vi "PDA_RegMode_Acquisition.vi"(4 "Shutter":bool=TRUE, 5 "error in":errorcluster, 6 "StartIng Mode":T1(ring)=enum."Reset", 7 "Number of Cycles":u32=1 min=1 max=30, 8 "Acquisition Parameters":T2={"Exposure (ms)"=100, "Interval (ms)"=10, "Flush Count"=1, "Trigger"=0} {"Trigger" items=["Disable", "Acquistion", "Cycle"]}) -> (0 "error out":errorcluster, 1 "# Pixel Overflow":i32, 2 "PDA Overflow":bool, 3 "Output Array":dbl[](array[numeric]) format="%.2f")   [LabVIEW 2019]
doc: "This VI demonstrates acquisition and image display of CCD data\nutilizing the ISA CCD driver.\n\nNote: Specific help is available for each individual control, display and indicator."
uses:
  Globals and TypeDefs/Type Definitions.llb/3 way Status.ctl
  Globals and TypeDefs/gStatus.vi
  IGA_comm.llb/Controller Version Number.vi
panel:
  out "PDA Temperature after":dbl
  out "Temperature":dbl
  in  "Tab Control":enum32{"Original Signals", "Averaged Output"}(tab)
  out "Display":sgl[][](graph)
  out "Display 2":dbl[](graph)
  out "Current Operation":T1(ring)
  in  "Gain":bool
  out "Read # count":u32=1 min=1 max=30
  in  "Number of Region copy":u32=4
  in  "Number of Regions":u32=1
  out "Acq Busy":bool
  # "Before        After"
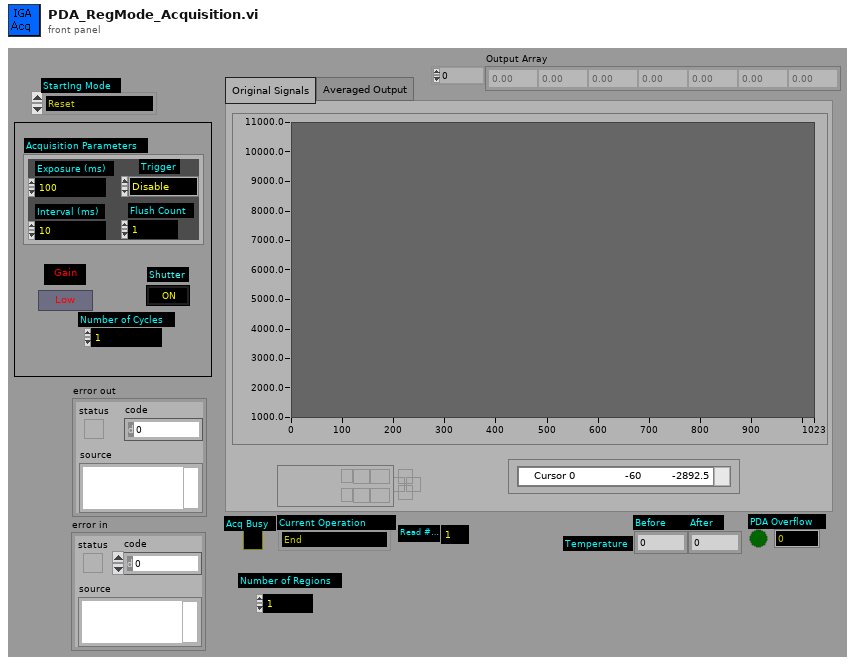
[diagram p1: front panel]
types:
  T1 = enum16{"End", "Init", "Reset", "SetAcqParameter", "SetArea", "Start Acquisition", "Busy Status Poll", "Read", "Stop"}
  T2 = cluster{"Exposure (ms)":u32, "Interval (ms)":u32, "Flush Count":i32, "Trigger":u16}
  T3 = typedef "3 way Status.ctl" = u8
  T4 = cluster{"Comm Interface":u16, "BUS":i16, "Address":i16, "Com Port":i32}
  T5 = enum16{"CCD Temperature Z345", "CCD Temperature Z308", "CCD Gain"}
  T6 = enum16{"Motor Init", "Motor Set Speed", "Motor Read Speed", "Motor Go", "Motor Busy Check", "Motor Move Relative", "Motor Set Position", "Motor Read Position", "Threshold Write Value", "Threshold Read Values", "Motor Limit Status", "Motor Stop", "ACQ Start", "ACQ Stop", "ACQ Integration Time Set", "ACQ Integration Time Read", "ACQ Busy", "ACQ Channel Gain Set", "ACQ Gain Read", "ACQ Read Data", "High Voltage Set", "High Voltage Read", "ACC Shutter Open", "ACC Shutter Close", "ACC Turret Position 1", "ACC Turret Position 0", "ACC ENTR Mirror Side", "ACC ENTR Mirror Front", "ACC Exit Mirror Side", "ACC Exit Mirror Front", "Slit Set Speed", "Slit Read Speed", "Slit Set Position", "Slit Read Position", "Slit Move Relative", "ACC Busy Check", "TTL Write Output", "TTL Read Output", "TTL Read Input", "Scan Set Parameters", "Scan Start", "Scan Current Status", "Scan Cycle to Read", "Scan Get Data Point Number", "Scan Get Data", "Scan Stop", "ACQ Measure Offsets", "ACQ Set Offsets", "TTL Automatic Outputs", "CCD_INIT", "CCD_SET_EXPOSURE_TIME", "CCD_SET_GAIN", "CCD_READ_GAIN", "CCD_SET_NUMBER_OF_FLUSHES", "CCD_SET_DOUBLE_COR_TIME", "CCD_SET_TEMPERATURE", "CCD_READ_TEMPERATURE", "CCD_READ_CHIP_STUFF", "CCD_START", "CCD_STATUS", "CCD_STOP", "CCD_READ_IMAGE", "CCD_READ_SCAN", "CCD_RESET_IMAGE", "CCD_READ_NEXT_SCAN", "CCD_RESET_SCAN", "CCD_SET_SHUTTER", "CCD_DEFINE_ACQ_FORMAT", "CCD_DEFINE_AREA", "CCD_GET_DATA_SIZE", "CCD_WRITE_CHIP_STUFF", "CCD_GO_BLAST", "CCD_TRIGGER_ENABLE", "CCD_SET_BLAST_INTERVAL", "CCD_WRITE_XDATA", "CCD_READ_XDATA", "CCD_STUFF_XDATA", "CCD_SET_MUX_AND_READ_ADC", "CCD_SET_SPEED_FACTOR", "CCD_SET_FLUSH_MODE", "CCD_GET_READOUT_TIME", "CCD Go ICCD", "CCD Select ADC"}
  T7 = cluster{"X Origin":u32, "Y Origin":u32, "X Size":u32, "Y Size":u32, "X Bin":u32, "Y Bin":u32}[]
  T8 = cluster{"Exposure (ms)":bool, "Interval (ms)":bool, "Flush Count":bool, "Trigger":bool}
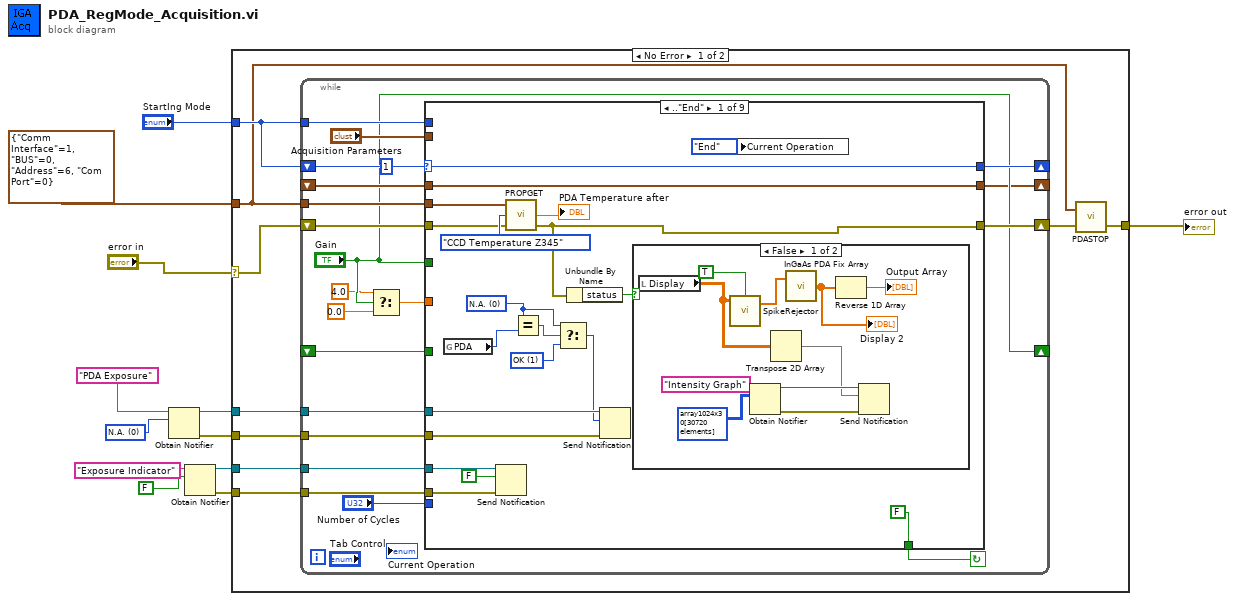
[diagram p0: block diagram]
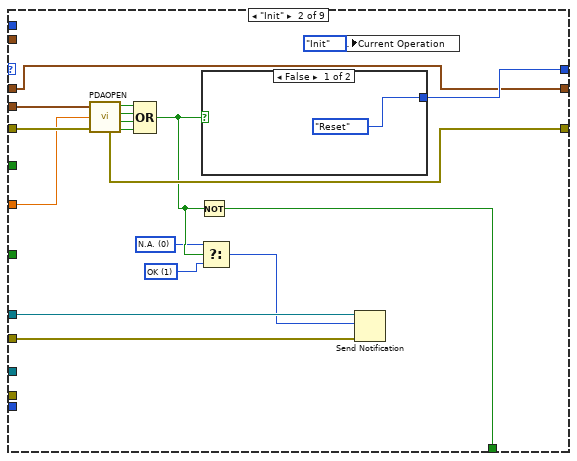
[diagram p3: hidden frame]
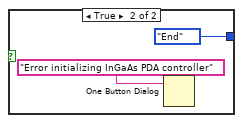
[diagram p4: hidden frame]
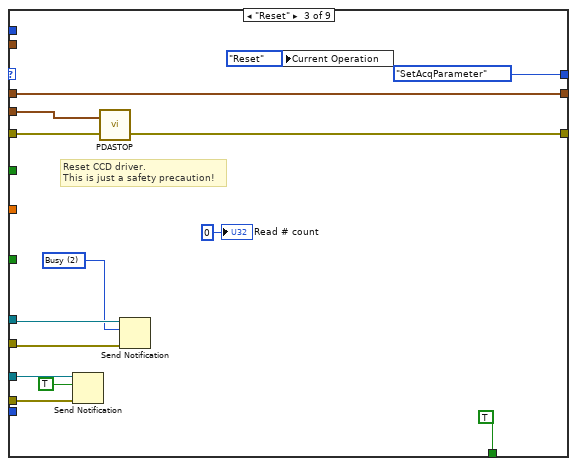
[diagram p5: hidden frame]
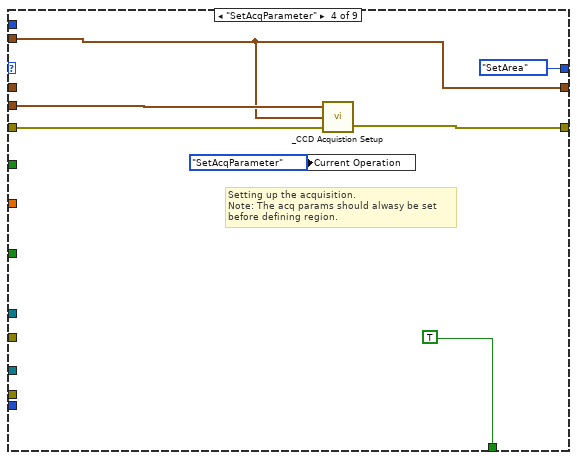
[diagram p6: hidden frame]
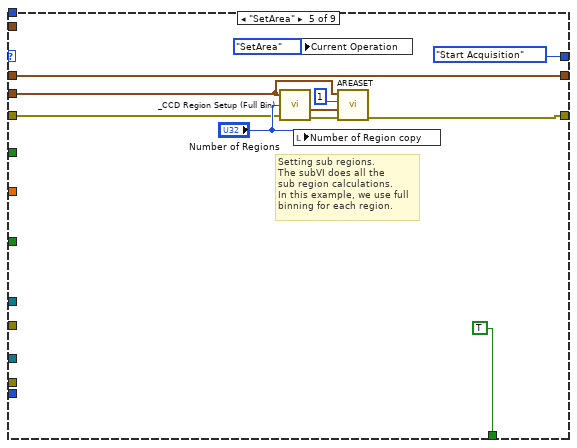
[diagram p7: hidden frame]
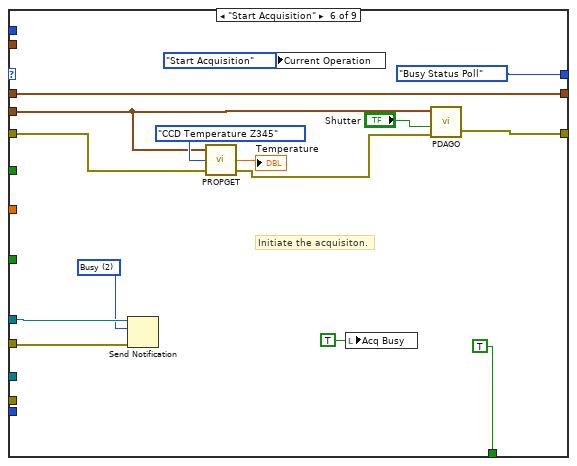
[diagram p8: hidden frame]
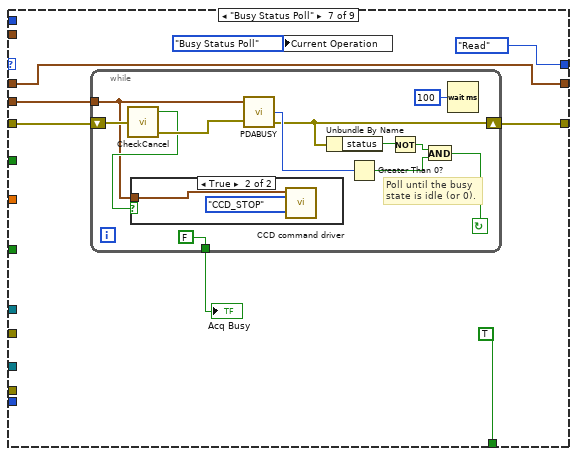
[diagram p9: hidden frame]
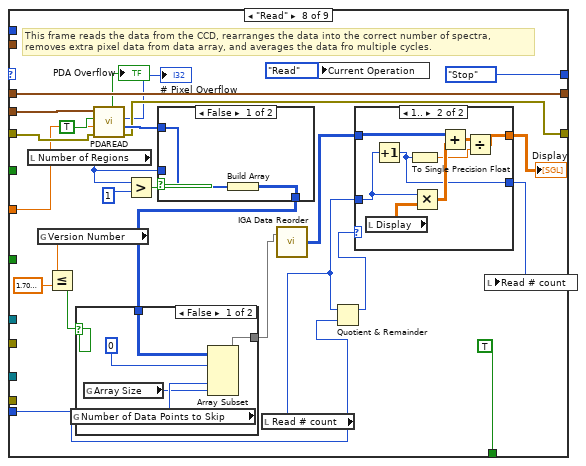
[diagram p11: hidden frame]
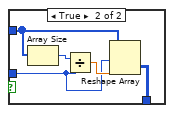
[diagram p13: hidden frame]
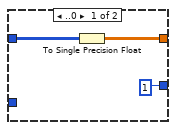
[diagram p14: hidden frame]
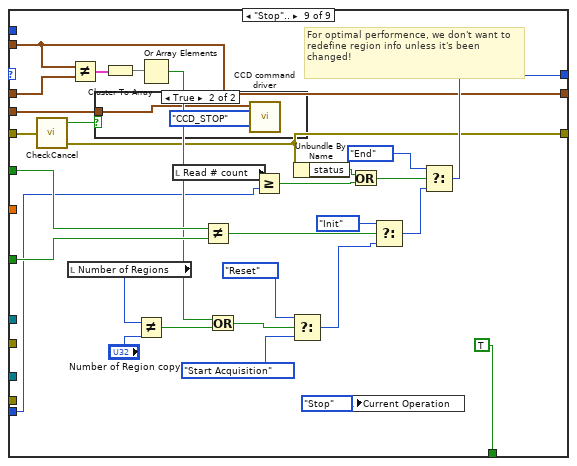
[diagram p15: hidden frame]
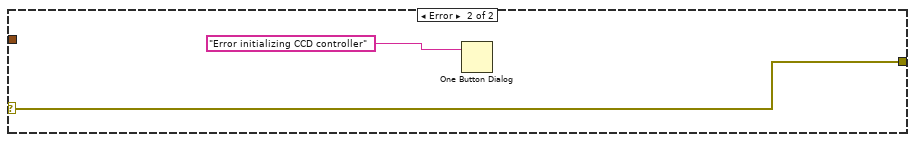
[diagram p17: hidden frame]
diagram:
  w8 = T3 0 items=["N.A.", "OK", "Busy", "Done"] ("Saving")
  n1 = Obtain Notifier(name (unnamed)="PDA Exposure", notification data type=w8) -> (notifier out=w7:refnum<notifier>, error out=w6:errorcluster)  [unwired: 2 in, 1 out]
  n2 = Obtain Notifier(name (unnamed)="Exposure Indicator", notification data type=FALSE ("SaveData?")) -> (notifier out=w3:refnum<notifier>, error out=w2:errorcluster)  [unwired: 2 in, 1 out]
  n3 = case shown="No Error" "error in" {
    selector: "error in" -> [w21 w244]
    tunnel: T4 {"Comm Interface"=1, "BUS"=0, "Address"=6, "Com Port"=0} ("Comm Params") -> [w17 _]
    tunnel: "StartIng Mode" -> [w19 _]
    tunnel: [w18 w244] -> w10
    tunnel: w7 -> [w16 _]
    tunnel: w6 -> [w15 _]
    tunnel: w3 -> [w14 _]
    tunnel: w2 -> [w13 _]
    frame No Error {
      (unwired) 1
      n4 = while {
        shift-left: w21 -> [w39]
        shift-right: [w40] -> w20
        tunnel: w17 -> [w38]
        shift-right: [w27] -> _
        shift-left: _ -> [w37]
        tunnel: w19 -> [w36]
        shift-right: ["Gain"] -> _
        shift-left: _ -> [w35]
        shift-right: [w34] -> _
        shift-left: w19 -> [w33]
        tunnel: w16 -> [w25]
        tunnel: w15 -> [w24]
        tunnel: w14 -> [w23]
        tunnel: w13 -> [w22]
        stop <- w41 continue-if-true
        n5 = Select(t=4.0, s="Gain", f=0.0) -> (s? t:f=w30:dbl)
        n6 = case shown="..\"End\"" w33 {
          selector: w33 -> [w60 _ _ _ _ _ _ _ _]
          tunnel: [FALSE w83 TRUE TRUE TRUE TRUE TRUE TRUE TRUE] -> w41
          tunnel: [w60 w81 T1."SetAcqParameter" ("StartIng Mode") T1."SetArea" ("StartIng Mode") T1."Start Acquisition" ("StartIng Mode") T1."Busy Status Poll" ("StartIng Mode") T1."Read" ("StartIng Mode") T1."Stop" ("StartIng Mode") w238] -> w34
          tunnel: w39 -> [w51 w85 w104 w111 w115 w127 w146 w170 w215]
          tunnel: [w49 w82 w103 w110 w118 w137 w144 w169 w214] -> w40
          tunnel: "Gain" -> [_ _ _ _ _ _ _ _ w234]
          tunnel: w38 -> [w50 w84 w102 w112 w119 w125 w145 w171 w212]
          tunnel: w37 -> [w59 w79 w101 _ w117 w134 w141 w166 w223]
          tunnel: w36 -> [_ _ _ _ _ _ _ _ _]
          tunnel: w35 -> [_ _ _ _ _ _ _ _ w233]
          tunnel: "Acquisition Parameters" -> [_ _ _ w108 _ _ _ _ w220]
          tunnel: w30 -> [_ w80 _ _ _ _ _ w167 _]
          tunnel: [w59 w79 w101 w108 w117 w134 w141 w166 w220] -> w27
          tunnel: "Number of Cycles" -> [_ _ _ _ _ _ _ w164 w217]
          tunnel: w25 -> [w57 w77 w98 _ _ w132 _ _ _]
          tunnel: w24 -> [w56 w76 w97 _ _ w131 _ _ _]
          tunnel: w23 -> [w44 _ w95 _ _ _ _ _ _]
          tunnel: w22 -> [w43 _ w94 _ _ _ _ _ _]
          frame .."End" {
            w45 = T3 0 items=["N.A.", "OK", "Busy", "Done"] ("x")
            w55 = T3 1 items=["N.A.", "OK", "Busy", "Done"] ("Saving")
            n7 = global read "gStatus.vi" "PDA"() -> (w47:T3)
            n8 = Send Notification(notification=FALSE, notifier=w44, error in (no error)=w43) -> ()  [unwired: 2 out]
            n9 = call "PROPGET.VI"("error in"=w51, "CCD Prop ID"=T5."CCD Temperature Z345", "Comm Params"=w50) -> ("error out"=w49:errorcluster, "Output Param"=→"PDA Temperature after":dbl)  [unwired: 1 out]
            n10 = Equal?(x=w45, y=w47) -> (x = y?=w46:bool)
            n11 = Select(t=w45, s=w46, f=w55) -> (s? t:f=w54:T3)
            n12 = Unbundle By Name(w49) -> ("status"=w48:bool)
            n13 = Send Notification(notification=w54, notifier=w57, error in (no error)=w56) -> ()  [unwired: 2 out]
            n14 = case shown="False" w48 {
              frame False {
                n15 = local read "Display"() -> (w63:sgl[][])
                n16 = call "SpikeRejector.vi"("Average Only (T)"=TRUE, "Input Array"=w63) -> ("Final Array"=w71:dbl[])  [unwired: 2 in, 1 out]
                n17 = Obtain Notifier(name (unnamed)="Intensity Graph", notification data type=i32[][] array1024x30[30720 elements] ("Intensity Graph")) -> (notifier out=w66:refnum<notifier>, error out=w67:errorcluster)  [unwired: 2 in, 1 out]
                n18 = Transpose 2D Array(2D array=w63) -> (transposed array=w62:sgl[][])
                n19 = call "InGaAs PDA Fix Array.vi"("Input Array"=w71) -> ("Output Array"=w69:dbl[])  [unwired: 2 in]
                "Display 2" <- w69
                n20 = Reverse 1D Array(array=w69) -> (reversed array=→"Output Array":dbl[])
                n21 = Send Notification(notification=w62, notifier=w66, error in (no error)=w67) -> ()  [unwired: 2 out]
              }
              frame True {
              }
            }
            n22 = local write "Current Operation"(T1."End" ("Current Operation")) -> ()
          }
          frame "Init" {
            w73 = T3 1 items=["N.A.", "OK", "Busy", "Done"] ("Saving")
            w74 = T3 0 items=["N.A.", "OK", "Busy", "Done"] ("Saving")
            n23 = call "PDAOPEN.VI"("error in"=w85, "CCD ADC and Gain"=w80, "Comm Params"=w84) -> ("State Error"=w86:bool, "error out"=w82:errorcluster, "Table Error"=w87:bool, "Init Error"=w88:bool, "Boot Error"=w89:bool)  [unwired: 1 out]
            n24 = Compound Arithmetic op=OR(w89, w88, w87, w86) -> (w75:bool)
            n25 = Not(x=w75) -> (.not. x?=w83:bool)
            n26 = Select(t=w74, s=w75, f=w73) -> (s? t:f=w72:T3)
            n27 = case shown="False" w75 {
              tunnel: [T1."Reset" ("StartIng Mode") T1."End" ("StartIng Mode")] -> w81
              frame False {
              }
              frame True {
                n28 = One Button Dialog(message="Error initializing InGaAs PDA controller") -> ()  [unwired: 1 in, 1 out]
              }
            }
            n29 = local write "Current Operation"(T1."Init" ("Current Operation")) -> ()
            n30 = Send Notification(notification=w72, notifier=w77, error in (no error)=w76) -> ()  [unwired: 2 out]
          }
          frame "Reset" {
            w96 = T3 2 items=["N.A.", "OK", "Busy", "Done"] ("notification")
            # "Reset CCD driver.\nThis is just a safety precaution!"
            n31 = Send Notification(notification=TRUE, notifier=w95, error in (no error)=w94) -> ()  [unwired: 2 out]
            n32 = call "PDASTOP.VI"("error in"=w104, "Comm Params"=w102) -> ("error out"=w103:errorcluster)  [unwired: 1 out]
            n33 = Send Notification(notification=w96, notifier=w98, error in (no error)=w97) -> ()  [unwired: 2 out]
            n34 = local write "Current Operation"(T1."Reset" ("Current Operation")) -> ()
            "Read # count" <- u32 0 ("Read count")
          }
          frame "SetAcqParameter" {
            # "Setting up the acquisition.\nNote: The acq params should alwasy be set\nbefore defining region."
            n35 = local write "Current Operation"(T1."SetAcqParameter" ("Current Operation")) -> ()
            n36 = call "_CCD Acquistion Setup.vi"("error in"=w111, "Acquisition Param"=w108, "Comm Params"=w112) -> ("error out"=w110:errorcluster)  [unwired: 1 out]
          }
          frame "SetArea" {
            # "Setting sub regions.\nThe subVI does all the\nsub region calculations.\nIn this example, we use full\nbinning for each region."
            n37 = call "_CCD Region Setup (Full Bin).vi"("Comm Params"=w119, "Number of Regions"="Number of Regions", "error in"=w115) -> ("Region Info Array"=w122:T7, "error out"=w114:errorcluster)  [unwired: 2 out]
            n38 = local write "Number of Region copy"("Number of Regions") -> ()
            n39 = local write "Current Operation"(T1."SetArea" ("Current Operation")) -> ()
            n40 = call "AREASET.VI"("error in"=w114, "Region Info Array"=w122, "Acquisition Format"=1, "Comm Params"=w119) -> ("error out"=w118:errorcluster)  [unwired: 3 in, 1 out]
          }
          frame "Start Acquisition" {
            w130 = T3 2 items=["N.A.", "OK", "Busy", "Done"] ("notification")
            # "Initiate the acquisiton."
            n41 = Send Notification(notification=w130, notifier=w132, error in (no error)=w131) -> ()  [unwired: 2 out]
            n42 = call "PROPGET.VI"("error in"=w127, "CCD Prop ID"=T5."CCD Temperature Z345", "Comm Params"=w125) -> ("error out"=w126:errorcluster, "Output Param"=→"Temperature":dbl)  [unwired: 1 out]
            n43 = local write "Current Operation"(T1."Start Acquisition" ("Current Operation")) -> ()
            n44 = local write "Acq Busy"(TRUE ("Acq Busy")) -> ()
            n45 = call "PDAGO.VI"("error in"=w126, "Shutter"="Shutter", "Comm Params"=w125) -> ("error out"=w137:errorcluster)  [unwired: 1 in, 1 out]
          }
          frame "Busy Status Poll" {
            n46 = while {
              shift-right: [w157] -> w144
              shift-left: w146 -> [w151]
              tunnel: w145 -> [w148]
              tunnel: [FALSE ("Acq Busy")] -> w142
              stop <- w153 continue-if-true
              # "Poll until the busy\nstate is idle (or 0)."
              n47 = call "CheckCancel.vi"("error in (no error)"=w151) -> ("Cancelled"=w149:bool, "error out"=w150:errorcluster)  [unwired: 1 in]
              n48 = case shown="True" w149 {
                tunnel: w148 -> [_ w160]
                frame False {
                }
                frame True {
                  n49 = call "CCD command driver.VI"("Command"=T6."CCD_STOP", "Comm Params"=w160) -> ()  [unwired: 5 in, 5 out]
                }
              }
              n50 = call "PDABUSY.VI"("Comm Params"=w148, "error in"=w150) -> ("CCD Status"=w159:u16, "error out"=w157:errorcluster)  [unwired: 1 out]
              n51 = Unbundle By Name(w157) -> ("status"=w156:bool)
              n52 = Greater Than 0?(x=w159) -> (x > 0?=w154:bool)
              n53 = Not(x=w156) -> (.not. x?=w155:bool)
              n54 = And(x=w155, y=w154) -> (x .and. y?=w153:bool)
              n55 = Wait (ms)(milliseconds to wait=u32 100) -> ()  [unwired: 1 out]
            }
            "Acq Busy" <- w142
            n56 = local write "Current Operation"(T1."Busy Status Poll" ("Current Operation")) -> ()
          }
          frame "Read" {
            # "This frame reads the data from the CCD, rearranges the data into the correct number of spectra, \nremoves extra pixel data from data array, and averages the data fro multiple cycles."
            n57 = local read "Number of Regions"() -> (w182:u32)
            n58 = global read "Controller Version Number.vi" "Version Number"() -> (w177:sgl)
            n59 = Less Or Equal?(x=w177, y=sgl 1.7) -> (x <= y?=w175:bool)
            n60 = call "PDAREAD.VI"("Comm Params"=w171, "Reset Image?"=TRUE, "CCD ADC and Gain"=w167, "error in"=w170) -> ("PDA Overflow"=→"PDA Overflow":bool, "Pixel Overflow"=→"# Pixel Overflow":i32, "Data"=w181:u16[], "error out"=w169:errorcluster)  [unwired: 1 out]
            n61 = Greater?(x=w182, y=u32 1) -> (0:w180:bool)
            n62 = case shown="False" w180 {
              tunnel: w181 -> [w194 w199]
              tunnel: [w195 w200] -> w174
              tunnel: w182 -> [_ w196]
              frame False {
                n63 = Build Array(w194) -> (w195:u16[][])
              }
              frame True {
                n64 = Array Size(array=w199) -> (size(s)=w198:i32)
                n65 = Divide(x=w198, y=w196) -> (x/y=w197:dbl)
                n66 = Reshape Array(w199, w196, w197) -> (w200:u16[][])
              }
            }
            n67 = case shown="False" w175 {
              tunnel: w174 -> [w192 w193]
              tunnel: [w191 w193] -> w173
              frame False {
                n68 = global read "Controller Version Number.vi" "Number of Data Points to Skip"() -> (w190:i8)
                n69 = global read "Controller Version Number.vi" "Array Size"() -> (w189:i32)
                n70 = Array Subset(array=w192, index (row)=0 ("Array Index"), index (col)=w190, length (col)=w189) -> (w191:u16[][])  [unwired: 1 in]
              }
              frame True {
              }
            }
            n71 = local read "Read # count"() -> (w184:u32)
            n72 = call "IGA Data Reorder.VI"("Input Array"=w173) -> ("Output Array"=w172:i32[][])  [unwired: 2 in]
            n73 = local write "Current Operation"(T1."Read" ("Current Operation")) -> ()
            n74 = Quotient & Remainder(x=w184, y=w164) -> (x-y*floor(x/y)=w186:u32)  [unwired: 1 out]
            n75 = case shown="1.." w186 {
              tunnel: w172 -> [w203 w210]
              tunnel: [w202 w206] -> w185
              tunnel: w184 -> [_ w205]
              tunnel: [u32 1 ("Read count") w204] -> w183
              frame ..0 {
                n76 = To Single Precision Float(number=w203) -> (single precision float=w202:sgl[][])
              }
              frame 1.. {
                n77 = local read "Display"() -> (w211:sgl[][])
                n78 = Increment(x=w205) -> (x+1=w204:u32)
                n79 = To Single Precision Float(number=w204) -> (single precision float=w207:sgl)
                n80 = Multiply(x=w205, y=w211) -> (x*y=w209:sgl[][])
                n81 = Add(x=w210, y=w209) -> (x+y=w208:sgl[][])
                n82 = Divide(x=w208, y=w207) -> (x/y=w206:sgl[][])
              }
            }
            "Display" <- w185
            n83 = local write "Read # count"(w183) -> ()
          }
          frame "Stop".. {
            # "For optimal performence, we don't want to redefine region info unless it's been changed!"
            n84 = call "CheckCancel.vi"("error in (no error)"=w215) -> ("Cancelled"=w213:bool, "error out"=w214:errorcluster)  [unwired: 1 in]
            n85 = local read "Number of Regions"() -> (w240:u32)
            n86 = Not Equal?(x=w220, y=w223) -> (x != y?=w225:T8)
            n87 = case shown="True" w213 {
              tunnel: w212 -> [_ w242]
              frame False {
              }
              frame True {
                n88 = call "CCD command driver.VI"("Command"=T6."CCD_STOP", "Comm Params"=w242) -> ()  [unwired: 5 in, 5 out]
              }
            }
            n89 = Cluster To Array(cluster=w225) -> (array=w224:bool[])
            n90 = Not Equal?(x=w240, y="Number of Region copy") -> (x != y?=w222:bool)
            n91 = Or Array Elements(Boolean array=w224) -> (logical OR=w226:bool)
            n92 = local read "Read # count"() -> (w218:u32)
            n93 = Not Equal?(x=w234, y=w233) -> (x != y?=w232:bool)
            n94 = Or(x=w226, y=w222) -> (x .or. y?=w221:bool)
            n95 = Greater Or Equal?(x=w218, y=w217) -> (x >= y?=w216:bool)
            n96 = Select(t=T1."Reset" ("StartIng Mode"), s=w221, f=T1."Start Acquisition") -> (s? t:f=w228:T1)
            n97 = Unbundle By Name(w214) -> ("status"=w236:bool)
            n98 = local write "Current Operation"(T1."Stop" ("Current Operation")) -> ()
            n99 = Or(x=w236, y=w216) -> (x .or. y?=w235:bool)
            n100 = Select(t=T1."Init" ("StartIng Mode"), s=w232, f=w228) -> (s? t:f=w227:T1)
            n101 = Select(t=T1."End" ("StartIng Mode"), s=w235, f=w227) -> (s? t:f=w238:T1)
          }
        }
      }
      n102 = call "PDASTOP.VI"("error in"=w20, "Comm Params"=w17) -> ("error out"=w18:errorcluster)  [unwired: 1 out]
    }
    frame Error {
      n103 = One Button Dialog(message="Error initializing CCD controller") -> ()  [unwired: 1 in, 1 out]
    }
  }
  "error out" <- w10
